vi "Barcode matching.vi"(6 "TFT WORNG SCANE":string="- TFT Barcode Scan Wrong", 8 "TFT BARCODE SCANE":string="- TFT Barcode Scan", 9 "Model":string, 10 "TFT Code":string, 11 "Serial data":string) -> (0 "Error":string, 1 "read buffer":string, 2 "result/trigger":bool, 3 "substring":string, 4 "Read bit":bool)   [LabVIEW 2015]
uses:
  Project Setup/Globle Variable/GR_Servo.vi
  Galobal variable_TI.vi
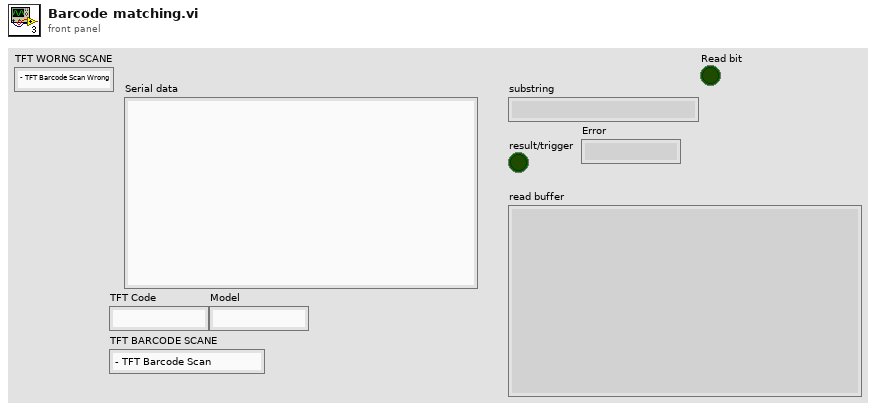
[diagram p1: front panel]
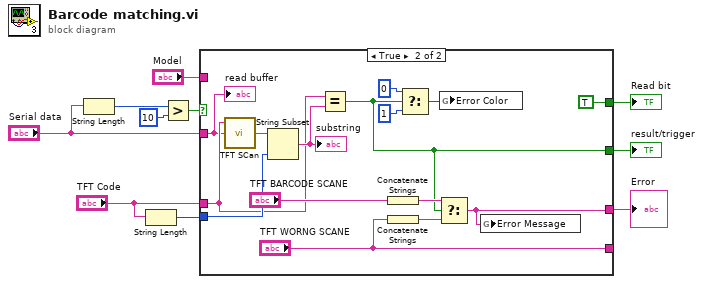
[diagram p0: block diagram]
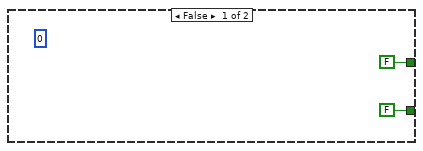
[diagram p2: hidden frame]
diagram:
  n1 = String Length(string="Serial data") -> (length=w6:i32)
  n2 = String Length(string="TFT Code") -> (length=w9:i32)
  n3 = Greater?(x=w6, y=10) -> (0:w8:bool)
  n4 = case shown="True" w8 {
    tunnel: "Serial data" -> [_ w14]
    tunnel: "TFT Code" -> [_ w15]
    tunnel: w9 -> [_ w27]
    tunnel: "Model" -> [_ _]
    tunnel: [FALSE w17] -> w2
    tunnel: [_ "TFT WORNG SCANE"] -> _
    tunnel: [_ w18] -> w3
    tunnel: [FALSE TRUE] -> w1
    frame False {
      (unwired) 0 ("f")
    }
    frame True {
      n5 = call "TFT SCan.vi"("Scan Data"=w14, "FTT"=w15) -> ("OutputData"=w13:string)  [unwired: 3 in]
      n6 = String Subset(string=w13, length (rest)=w27) -> (substring=w26:string)  [unwired: 1 in]
      "substring" <- w26
      n7 = Equal?(x=w15, y=w26) -> (x = y?=w17:bool)
      n8 = Concatenate Strings("TFT BARCODE SCANE") -> (w22:string)
      n9 = Concatenate Strings("TFT WORNG SCANE") -> (w21:string)
      n10 = Select(t=0, s=w17, f=1) -> (s? t:f=w19:i32)
      n11 = Select(t=w22, s=w17, f=w21) -> (s? t:f=w18:string)
      n12 = global write "Galobal variable_TI.vi" "Error Color"(w19) -> ()
      n13 = global write "GR_Servo.vi" "Error Message"(w18) -> ()
      "read buffer" <- w14
    }
  }
  "Error" <- w3
  "result/trigger" <- w2
  "Read bit" <- w1
